vi "add_text.vi"(8 "error in (no error)":errorcluster, 10 "string in":string, 11 "new string":string) -> (0 "error out":errorcluster, 3 "string out":string)   [LabVIEW 2015]
doc: "adds a \"new string\" to the existing \"string in\".\nA linefeed/carriage return is added to the \"string in\" first."
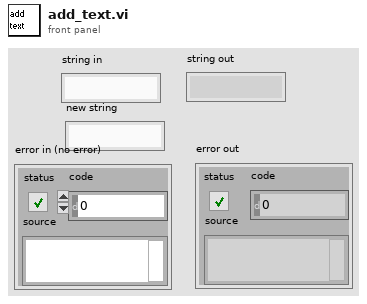
[diagram p1: front panel]
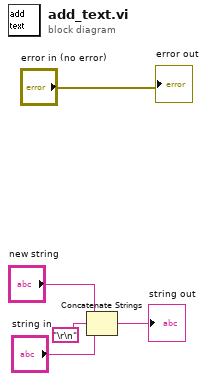
[diagram p0: block diagram]
diagram:
  n1 = Concatenate Strings("new string", "\r\n", "string in") -> (→"string out":string)
  "error out" <- "error in (no error)"
